vi "getError.vi"() -> (0 "error out":errorcluster)   [LabVIEW 2014]
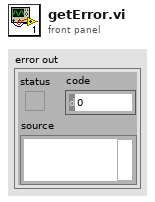
[diagram p1: front panel]
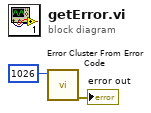
[diagram p0: block diagram]
diagram:
  n1 = call <vilib>:"Error Cluster From Error Code.vi"("error code (0)"=1026) -> ("error out"=→"error out":errorcluster)  [unwired: 8 in]
